vi "configuration_to_runtime.vi"(8 "error in (no error)":errorcluster, 11 "configuration":T3) -> (0 "error out":errorcluster, 3 "runtime":T1={"tag_name"="", "type"="<type>", "offset"=0.0, "slope"=0.0, "formula"="", "x_points"=[], "y_points"=[]})   [LabVIEW 2015, in "lv-calibration.lvlib"]
uses:
  lv-calibration.lvlib
  <userlib>/antonio-alexander/lv-calibration/public/_controls/configuration.ctl
  _controls/type.ctl
  <userlib>/antonio-alexander/lv-calibration/public/_controls/point.ctl
  _controls/runtime.ctl
  _controls/error.ctl
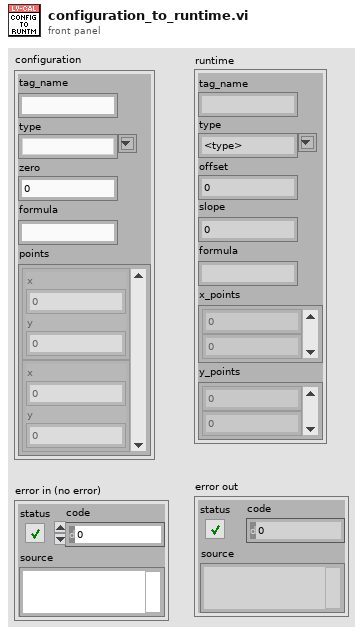
[diagram p1: front panel]
types:
  T1 = typedef "lv-calibration.lvlib/runtime.ctl" = cluster{"tag_name":string, "type":T2, "offset":dbl, "slope":dbl, "formula":string, "x_points":dbl[], "y_points":dbl[]}
  T2 = typedef "lv-calibration.lvlib/type.ctl" = string
  T3 = typedef "configuration.ctl" = cluster{"tag_name":string, "type":T2, "zero":dbl, "formula":string, "points":T4[]}
  T4 = typedef "point.ctl" = cluster{"x":dbl, "y":dbl}
  T5 = typedef "lv-calibration.lvlib/error.ctl" = enum16{"<error>", "unsupported_calibration_type", "tag_name_not_found", "duplicate_tag_names", "formula_empty"}
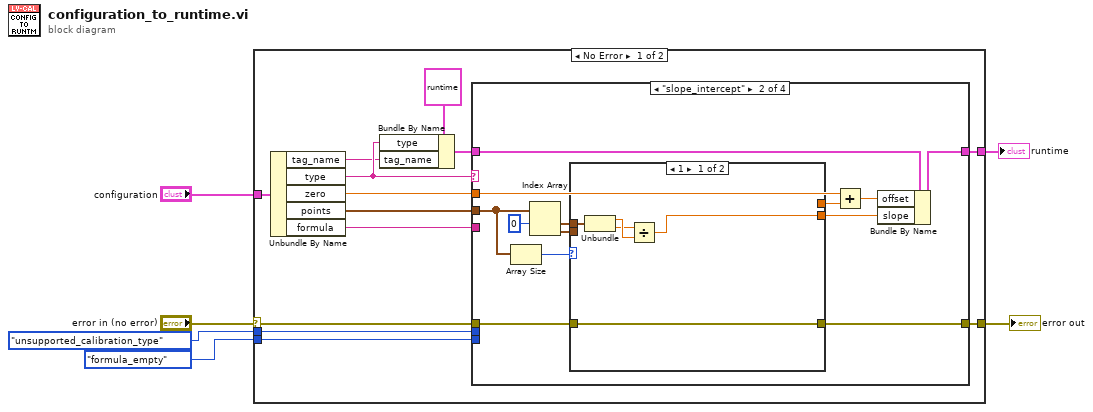
[diagram p0: block diagram]
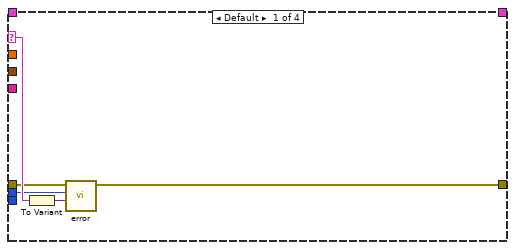
[diagram p2: hidden frame]
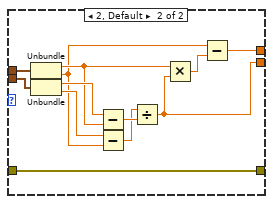
[diagram p3: hidden frame]
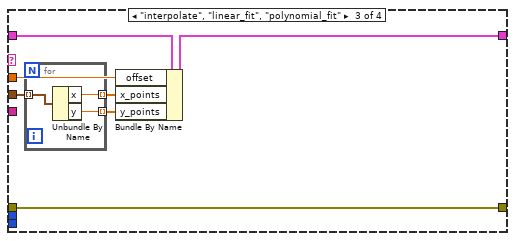
[diagram p4: hidden frame]
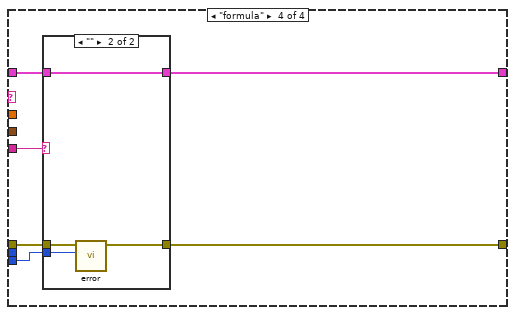
[diagram p5: hidden frame]
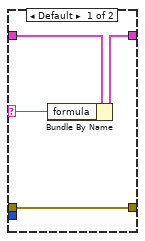
[diagram p6: hidden frame]
diagram:
  n1 = case shown="No Error" "error in (no error)" {
    selector: "error in (no error)" -> [w15 w79]
    tunnel: "configuration" -> [w19 _]
    tunnel: [w14 w79] -> w4
    tunnel: [w13 _] -> w3
    tunnel: error."unsupported_calibration_type" ("error") -> [w10 _]
    tunnel: error."formula_empty" ("error") -> [w8 _]
    frame No Error {
      n2 = Unbundle By Name(w19) -> ("tag_name"=w7:string, "type"=w11:T2, "zero"=w18:dbl, "points"=w17:T4[], "formula"=w9:string)
      n3 = Bundle By Name(cluster=T1 {"tag_name"="", "type"="<type>", "offset"=0.0, "slope"=0.0, "formula"="", "x_points"=[], "y_points"=[]}, "type"=w11, "tag_name"=w7) -> (w12:T1)
      n4 = case shown="\"slope_intercept\"" w11 {
        selector: w11 -> [w24 _ _ _]
        tunnel: w18 -> [_ w36 w59 _]
        tunnel: w17 -> [_ w25 w57 _]
        tunnel: w12 -> [_ w37 w61 w66]
        tunnel: w15 -> [w23 w33 w60 w69]
        tunnel: [w22 w28 w60 w67] -> w14
        tunnel: [_ w29 w58 w65] -> w13
        tunnel: w10 -> [w21 _ _ _]
        tunnel: w9 -> [_ _ _ w70]
        tunnel: w8 -> [_ _ _ w68]
        frame Default {
          n5 = To Variant(anything=w24) -> (Variant=w20:variant)
          n6 = call "error.vi"("data"=w20, "error"=w21, "error in (no error)"=w23) -> ("error out"=w22:errorcluster)  [unwired: 8 in]
        }
        frame "slope_intercept" {
          n7 = Array Size(array=w25) -> (size(s)=w34:i32)
          n8 = Index Array(array=w25, index #1=0 ("index")) -> (element #1=w32:T4, element #2=w31:T4)  [unwired: 1 in]
          n9 = case shown="1" w34 {
            tunnel: w32 -> [w42 w54]
            tunnel: w33 -> [w38 w44]
            tunnel: w31 -> [_ w53]
            tunnel: [w38 w44] -> w28
            tunnel: [w39 w49] -> w27
            tunnel: [_ w45] -> w26
            frame 1 {
              n10 = Unbundle(w42) -> ("x"=w41:dbl, "y"=w40:dbl)
              n11 = Divide(x=w40, y=w41) -> (x/y=w39:dbl)
            }
            frame 2, Default {
              n12 = Unbundle(w54) -> ("x"=w48:dbl, "y"=w43:dbl)
              n13 = Unbundle(w53) -> ("x"=w52:dbl, "y"=w46:dbl)
              n14 = Subtract(x=w52, y=w48) -> (x-y=w51:dbl)
              n15 = Subtract(x=w46, y=w43) -> (x-y=w50:dbl)
              n16 = Divide(x=w50, y=w51) -> (x/y=w49:dbl)
              n17 = Multiply(x=w48, y=w49) -> (x*y=w47:dbl)
              n18 = Subtract(x=w43, y=w47) -> (x-y=w45:dbl)
            }
          }
          n19 = Add(x=w36, y=w26) -> (x+y=w35:dbl)
          n20 = Bundle By Name(cluster=w37, "offset"=w35, "slope"=w27) -> (w29:T1)
        }
        frame "interpolate", "linear_fit", "polynomial_fit" {
          n21 = for {
            tunnel: w57 -> [w64] mode=indexing
            tunnel: [w63] -> w56 mode=indexing
            tunnel: [w62] -> w55 mode=indexing
            n22 = Unbundle By Name(w64) -> ("x"=w63:dbl, "y"=w62:dbl)
          }
          n23 = Bundle By Name(cluster=w61, "offset"=w59, "x_points"=w56, "y_points"=w55) -> (w58:T1)
        }
        frame "formula" {
          n24 = case shown="\"\"" w70 {
            selector: w70 -> [w73 _]
            tunnel: w69 -> [w71 w78]
            tunnel: w68 -> [_ w77]
            tunnel: [w71 w76] -> w67
            tunnel: w66 -> [w74 w75]
            tunnel: [w72 w75] -> w65
            frame Default {
              n25 = Bundle By Name(cluster=w74, "formula"=w73) -> (w72:T1)
            }
            frame "" {
              n26 = call "error.vi"("error"=w77, "error in (no error)"=w78) -> ("error out"=w76:errorcluster)  [unwired: 9 in]
            }
          }
        }
      }
    }
    frame Error {
    }
  }
  "error out" <- w4
  "runtime" <- w3
